vi "Add Alarm.vi"(7 "Overwrite Existing?":bool=TRUE, 8 "error in (no error)":errorcluster, 9 "Alarm Settings":T1={"Name"="", "Description"="", "Alarm Channel Node Path"="", "UpperLimit"=0.0, "Upper Limit Channel Node Path"="", "LowerLimit"=0.0, "Lower Limit Channel Node Path"="", "Alarm Action Node Path"="", "Mode"=0, "DefaultState"=1, "Priority"=0, "Delay"=0.0, "TripMessage"="", "GroupNumber"=0} {"Priority" items=["Low", "Medium", "High"]; "DefaultState" items=["Disabled", "Enabled"]; "Mode" items=["Normal", "IndicateOnly"]}, 10 "Base Node Path":string, 11 "SysDef Ref":T2) -> (0 "error out":errorcluster, 2 "New Node Path":string, 3 "SysDef Ref Out":T2)   [LabVIEW 2019, in "Simple SysDef API.lvlib"]
uses:
  <userlib>/SimpleSysDef/Simple SysDef API.lvlib
  <userlib>/SimpleSysDef/_SubVIs/System Definition Reference.ctl
  NationalInstruments.VeriStand.SystemDefinitionAPI
  <userlib>/SimpleSysDef/_SubVIs/Add Alarm_Settings.ctl
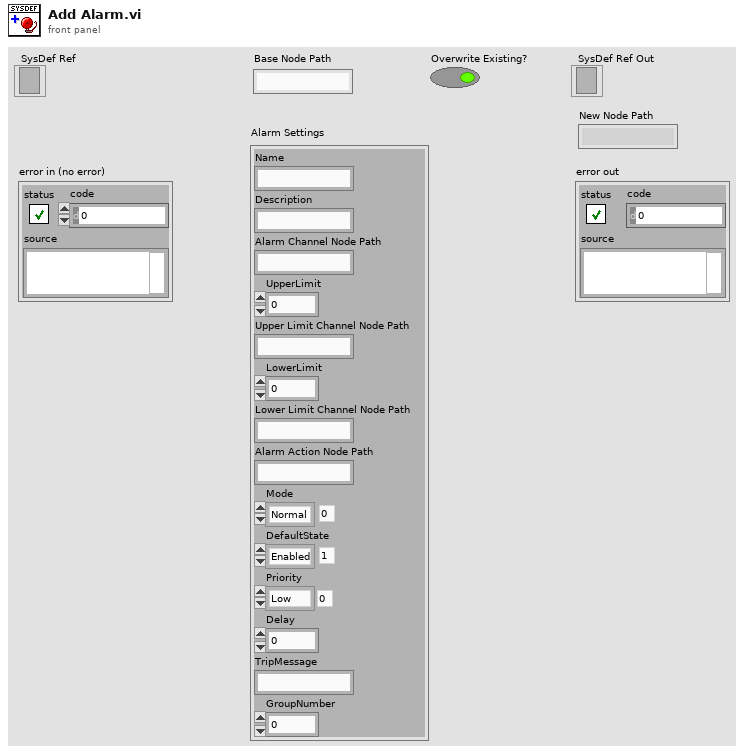
[diagram p1: front panel]
types:
  T1 = typedef "Simple SysDef API.lvlib/Add Alarm_Settings.ctl" = cluster{"Name":string, "Description":string, "Alarm Channel Node Path":string, "UpperLimit":dbl, "Upper Limit Channel Node Path":string, "LowerLimit":dbl, "Lower Limit Channel Node Path":string, "Alarm Action Node Path":string, "Mode":i32, "DefaultState":i32, "Priority":i32, "Delay":dbl, "TripMessage":string, "GroupNumber":u32}
  T2 = typedef "Simple SysDef API.lvlib/System Definition Reference.ctl" = refnum<k24>
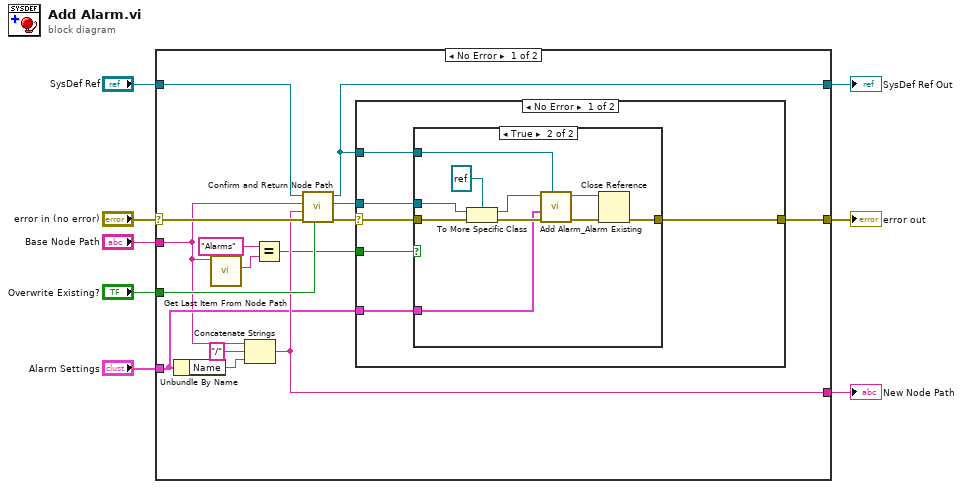
[diagram p0: block diagram]
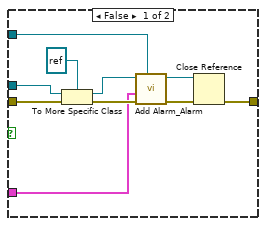
[diagram p2: hidden frame]
diagram:
  n1 = case shown="No Error" "error in (no error)" {
    selector: "error in (no error)" -> [w23 w52]
    tunnel: [w19 w52] -> w7
    tunnel: "SysDef Ref" -> [w22 w51]
    tunnel: [w14 w51] -> w5
    tunnel: "Base Node Path" -> [w10 _]
    tunnel: "Overwrite Existing?" -> [w16 _]
    tunnel: "Alarm Settings" -> [w13 _]
    tunnel: [w15 _] -> w1
    frame No Error {
      n2 = Unbundle By Name(w13) -> ("Name"=w20:string)
      n3 = call <userlib>:"Get Last Item From Node Path.vi"("Name"=w10) -> ("Last Item"=w11:string)  [unwired: 9 in, 1 out]
      n4 = Concatenate Strings(w10, "/" ("string"), w20) -> (w15:string)
      n5 = Equal?(x="Alarms", y=w11) -> (x = y?=w9:bool)
      n6 = call <userlib>:"Confirm and Return Node Path.vi"("Overwrite Existing?"=w16, "error in (no error)"=w23, "New Node Path"=w15, "Base Node Path"=w10, "SysDef Ref"=w22) -> ("error out"=w17:errorcluster, "Node Ref"=w18:refnum<k24>, "SysDef Ref Out"=w14:T2)  [unwired: 4 in]
      n7 = case shown="No Error" w17 {
        selector: w17 -> [w28 w50]
        tunnel: [w27 w50] -> w19
        tunnel: w18 -> [w29 _]
        tunnel: w14 -> [w26 _]
        tunnel: w13 -> [w25 _]
        tunnel: w9 -> [w24 _]
        frame No Error {
          n8 = case shown="True" w24 {
            tunnel: w29 -> [w39 w49]
            tunnel: w28 -> [w38 w48]
            tunnel: [w37 w47] -> w27
            tunnel: w26 -> [w31 w42]
            tunnel: w25 -> [w30 w44]
            frame False {
              n9 = To More Specific Class(target class=refnum<k24> refnum ("Node Ref"), reference=w39, error in=w38) -> (specific class reference=w35:refnum<k24>, error out=w33:errorcluster)
              n10 = call <userlib>:"Add Alarm_Alarm.vi"("SysDef Ref"=w31, "error in (no error)"=w33, "Alarm Settings"=w30, "Alarm Folder Ref"=w35) -> ("error out"=w32:errorcluster, "Alarm Folder Ref out"=w34:refnum<k24>)  [unwired: 6 in]
              n11 = Close Reference(reference=w34, error in (no error)=w32) -> (error out=w37:errorcluster)
            }
            frame True {
              n12 = To More Specific Class(target class=refnum<k24> refnum ("Node Ref"), reference=w49, error in=w48) -> (specific class reference=w43:refnum<k24>, error out=w45:errorcluster)
              n13 = call <userlib>:"Add Alarm_Alarm Existing.vi"("SysDef Ref"=w42, "error in (no error)"=w45, "Alarm Settings"=w44, "Alarm Folder Ref"=w43) -> ("error out"=w40:errorcluster, "Alarm Folder Ref out"=w41:refnum<k24>)  [unwired: 6 in]
              n14 = Close Reference(reference=w41, error in (no error)=w40) -> (error out=w47:errorcluster)
            }
          }
        }
        frame Error {
        }
      }
    }
    frame Error {
    }
  }
  "SysDef Ref Out" <- w5
  "error out" <- w7
  "New Node Path" <- w1
